vi "sub parse frame b.vi"(8 "error in (no error)":errorcluster, 11 "<b> String":string="<b kind 0 x 21 y 24 w 42 h 60 b>") -> (0 "error out":errorcluster, 3 "<b> data":T1)   [LabVIEW 2018, in "Data Parser.lvclass"]
uses:
  Data Parser.lvclass
  frame b data.ctl
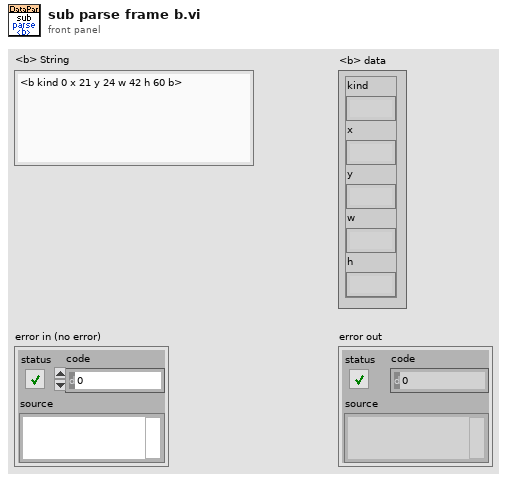
[diagram p1: front panel]
types:
  T1 = typedef "Data Parser.lvclass/frame b data.ctl" = cluster{"kind":string, "x":string, "y":string, "w":string, "h":string}
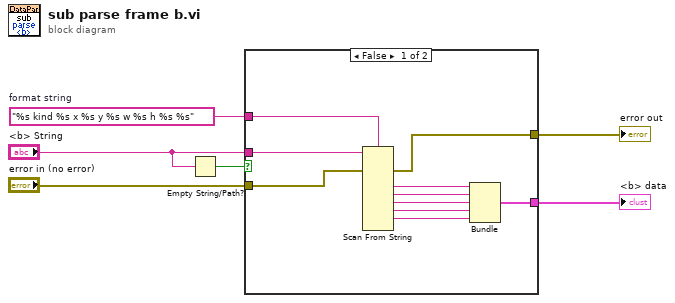
[diagram p0: block diagram]
diagram:
  w6 = "%s kind %s x %s y %s w %s h %s %s"  # format string
  n1 = Empty String/Path?(string/path="<b> String") -> (empty?=w1:bool)
  n2 = case shown="False" w1 {
    tunnel: "<b> String" -> [w16 _]
    tunnel: w6 -> [w15 _]
    tunnel: [w12 _] -> w5
    tunnel: "error in (no error)" -> [w11 w17]
    tunnel: [w10 w17] -> w3
    frame False {
      n3 = Scan From String(format string=w15, input string=w16, error in=w11) -> (error out=w10:errorcluster, output 2=w14:string, output 3=w13:string, output 4=w9:string, output 5=w8:string, output 6=w7:string)  [unwired: 10 in, 2 out]
      n4 = Bundle(w14, w13, w9, w8, w7) -> (w12:cluster{string, string, string, string, string})  [unwired: 1 in]
    }
    frame True {
    }
  }
  "<b> data" <- w5
  "error out" <- w3
